vi "ExposeInvokeParamterRemoteValueUpdateEvent.vi"(8 "Invoke Value Labview Value Update event":bool, 9 "Names":string[](array[string]), 10 "Name":string, 11 "Expose Info":T1) -> ()   [LabVIEW 2017]
uses:
  Core/ExposeInfo.ctl
  C:/Code/CMCryoSysCode/Expose/COM/CSCom/CSCom/bin/Release/CSCom.dll
  COM/CSCom/CSCom/bin/Release/CSCom.dll
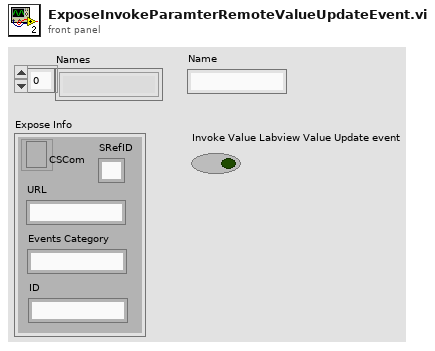
[diagram p1: front panel]
types:
  T1 = typedef "ExposeInfo.ctl" = cluster{"CSCom":refnum<k24>, "URL":string, "Events Category":string, "ID":string, "SRefID":string}
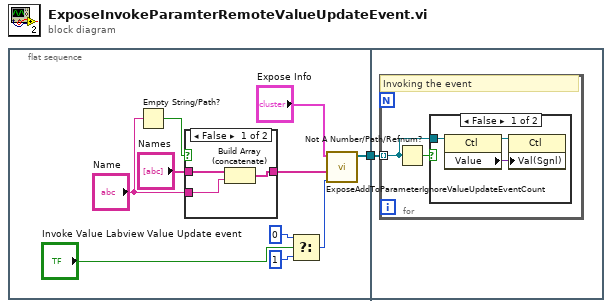
[diagram p0: block diagram]
diagram:
  n1 = flat-sequence {
    tunnel: [w6] -> w1
    tunnel: w1 -> [w16]
    frame #0 {
      n2 = Empty String/Path?(string/path="Name") -> (empty?=w11:bool)
      n3 = case shown="False" w11 {
        tunnel: "Names" -> [w13 w15]
        tunnel: "Name" -> [w14 _]
        tunnel: [w12 w15] -> w7
        frame False {
          n4 = Build Array (concatenate)(w13, w14) -> (w12:string[])
        }
        frame True {
        }
      }
      n5 = Select(t=0, s="Invoke Value Labview Value Update event", f=1 ("Add to count (0)")) -> (s? t:f=w2:i32)
      n6 = call "ExposeAddToParameterIgnoreValueUpdateEventCount.vi"("Add to count (0)"=w2, "Names"=w7, "Expose Info"="Expose Info") -> ("Updated Controls"=w6:refnum<vi>[])  [unwired: 8 in]
    }
    frame #1 {
      n7 = for {
        tunnel: w16 -> [w17] mode=indexing
        # "Invoking the event"
        n8 = Not A Number/Path/Refnum?(number/path/refnum=w17) -> (NaN/Path/Refnum?=w18:bool)
        n9 = case shown="False" w18 {
          tunnel: w17 -> [w20 _]
          frame False {
            n10 = property class="Ctl"(reference=w20) -> (reference out=w19:refnum<vi>, "Value"=w21:variant)  [unwired: 1 in, 1 out]
            n11 = property class="Ctl"(reference=w19, "Val(Sgnl)"=w21) -> ()  [unwired: 1 in, 2 out]
          }
          frame True {
          }
        }
      }
    }
  }
